vi "SPARK Get Signal Config.vi"   [LabVIEW 2023]
doc: "Get the configuration of a specific signal of the SPARK."
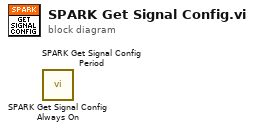
[diagram p0: block diagram]
diagram:
  n1 = call "SPARK Get Signal Config Always On.vi"() -> ()  [unwired: 9 in, 3 out]
  n2 = call "SPARK Get Signal Config Period.vi"() -> ()  [unwired: 9 in, 3 out]
